vi "Simulate Signal.vi"() -> ()   [LabVIEW 2023]
panel:
  in  "?":bool
  out "Waveform Chart":dynamicdata(graph)
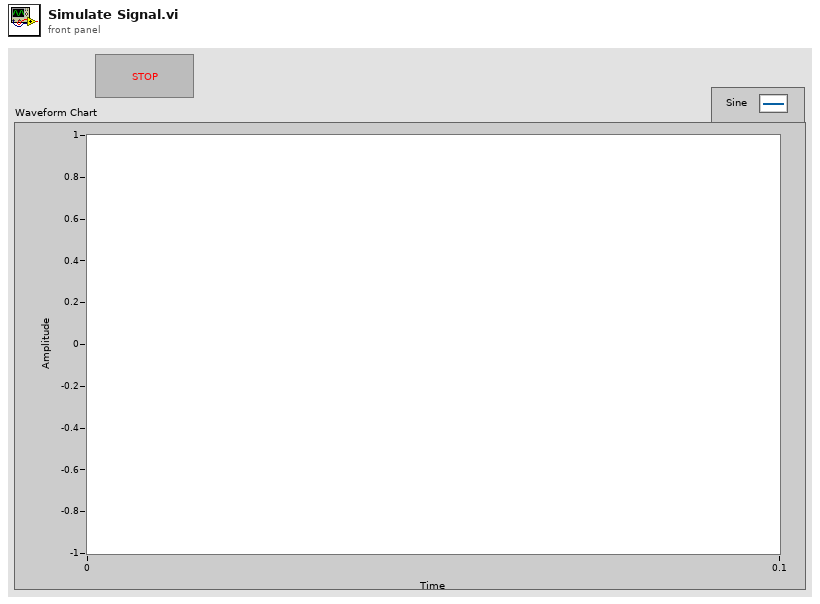
[diagram p1: front panel]
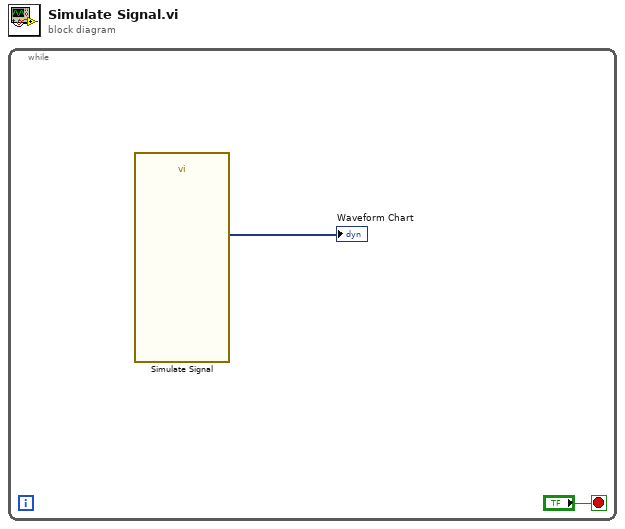
[diagram p0: block diagram]
diagram:
  n1 = while {
    stop <- "?" stop-if-true
    n2 = call "Simulate Signal"() -> ("Sine"=→"Waveform Chart":dynamicdata)  [unwired: 14 in, 1 out]
  }
